vi "USBClient2Pub.vi"() -> ()   [LabVIEW 2018]
uses:
  <vilib>/daq.io/MQTT LabVIEW Client/Controls/Connect_Flags.ctl
  <vilib>/daq.io/MQTT LabVIEW Client/Controls/QoS.ctl
  <vilib>/daq.io/MQTT LabVIEW Client/Controls/DUP_Flag.ctl
  <vilib>/daq.io/MQTT LabVIEW Client/Controls/Retain_Flag.ctl
  <vilib>/DAQmx/read.llb/DAQmx Read (Analog DBL 1Chan 1Samp).vi
  <vilib>/DAQmx/create/channels.llb/DAQmx Create Channel (AI-Voltage-Basic).vi
  <vilib>/DAQmx/miscellaneous.llb/DAQmx Fill In Error Info.vi
  <vilib>/daq.io/MQTT LabVIEW Client/MQTT_Functions.lvlib
panel:
  out "Temperature":dbl format="%#_3g"
  in  "stop":bool
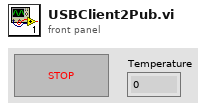
[diagram p1: front panel]
types:
  T1 = typedef "MQTT_Functions.lvlib/QoS.ctl" = enum8{"At most once", "At least once", "Exactly once", "Reserved"}
  T2 = typedef "MQTT_Functions.lvlib/Retain_Flag.ctl" = bool
  T3 = typedef "MQTT_Functions.lvlib/DUP_Flag.ctl" = bool
  T4 = cluster{"QoS":T1, "DUP":T3, "Retain":T2, "Keep Alive (sec)":u16}
  T5 = typedef "MQTT_Functions.lvlib/Connect_Flags.ctl" = cluster{"user name":bool, "password":bool, "will retain":bool, "will flag":bool, "clean session":bool, "reserved":bool, "will QoS":T1}
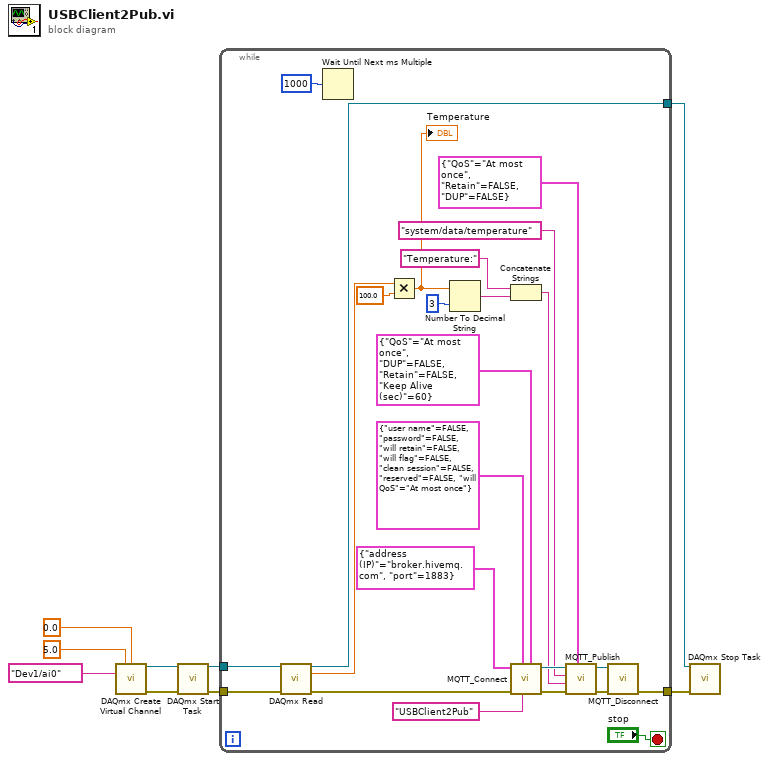
[diagram p0: block diagram]
diagram:
  n1 = call-poly <vilib>:"DAQmx Create Virtual Channel.vi"("maximum value"=5.0, "minimum value"=0.0, "physical channels"=tag "Dev1/ai0") -> ("task out"=w6:refnum<k21>, "error out"=w5:errorcluster)  [unwired: 11 in]
  n2 = call <vilib>:"DAQmx Start Task.vi"("task/channels in"=w6, "error in"=w5) -> ("task out"=w4:refnum<k21>, "error out"=w3:errorcluster)  [unwired: 12 in]
  n3 = while {
    tunnel: w4 -> [w33]
    tunnel: w3 -> [w32]
    tunnel: [w31] -> w2
    tunnel: [w13] -> w1
    stop <- "stop" stop-if-true
    n4 = call-poly <vilib>:"DAQmx Read.vi"("task/channels in"=w33, "error in"=w32) -> ("task out"=w31:refnum<k21>, "data"=w12:dbl, "error out"=w30:errorcluster)  [unwired: 11 in]
    n5 = Wait Until Next ms Multiple(millisecond multiple=u32 1000) -> ()  [unwired: 1 out]
    n6 = Multiply(x=w12, y=100.0) -> (x*y=w10:dbl)
    "Temperature" <- w10
    n7 = Number To Decimal String(number=w10, width (-)=i16 3) -> (decimal integer string=w19:string)
    n8 = Concatenate Strings("Temperature:" ("Message to be published"), w19) -> (w21:string)
    n9 = call <vilib>:"MQTT_Connect.vi"("Connect Meta"=T4 {"QoS"=enum."At most once", "DUP"=FALSE, "Retain"=FALSE, "Keep Alive (sec)"=60}, "Client ID"="USBClient2Pub", "Connect Flags"=T5 {"user name"=FALSE, "password"=FALSE, "will retain"=FALSE, "will flag"=FALSE, "clean session"=FALSE, "reserved"=FALSE, "will QoS"=enum."At most once"}, "error in (no error)"=w30, "MQTT Broker"=cluster{"address (IP)":string, "port":u16} {"address (IP)"="broker.hivemq.com", "port"=1883}) -> ("error out"=w25:errorcluster, "connection ID out"=w24:refnum<k5>)  [unwired: 4 in, 1 out]
    n10 = call <vilib>:"MQTT_Publish.vi"("Publish Meta"=cluster{"QoS":T1, "Retain":T2, "DUP":T3} {"QoS"=enum."At most once", "Retain"=FALSE, "DUP"=FALSE}, "error in (no error)"=w25, "Message to be published"=w21, "Topic"="system/data/temperature", "connection ID"=w24) -> ("error out"=w16:errorcluster, "connection ID out"=w17:refnum<k5>)  [unwired: 5 in]
    n11 = call <vilib>:"MQTT_Disconnect.vi"("error in (no error)"=w16, "connection ID"=w17) -> ("error out"=w13:errorcluster)  [unwired: 9 in]
  }
  n12 = call <vilib>:"DAQmx Stop Task.vi"("task/channels in"=w2, "error in"=w1) -> ()  [unwired: 12 in, 2 out]
